vi "Idot Continuous Recorder.vi"(8 "Error In":errorcluster, 9 "New data file event":refnum<user-event>, 10 "Stop event":refnum<user-event>, 11 "Parameters":T1={"physical channels"="Dev1/ai0:7", "input terminal configuration"=10106, "Range"=10.0, "Sample rate"=1000000.0, "samples per channel"=220000, "Trigger source"="/Dev1/PFI0", "pretrigger samples per channel"=20000, "task"="", "Sample mode"=10178, "Retriggerable"=FALSE, "File Path"=path ""} {"Sample mode" items=["Finite Samples"=10178, "Continuous Samples"=10123, "Hardware Timed Single Point"=12522]; "Sample rate" format="%.2p"; "input terminal configuration" items=["default"=-1, "RSE"=10083, "NRSE"=10078, "Differential"=10106, "Pseudodifferential"=12529]}) -> (0 "Error Out":errorcluster)   [LabVIEW 2015]
uses:
  NI-DAQ/NI-DAQ digitizer parameters.ctl
  <resource>/objmgr/daqmx.rc
panel:
  out "Done":bool
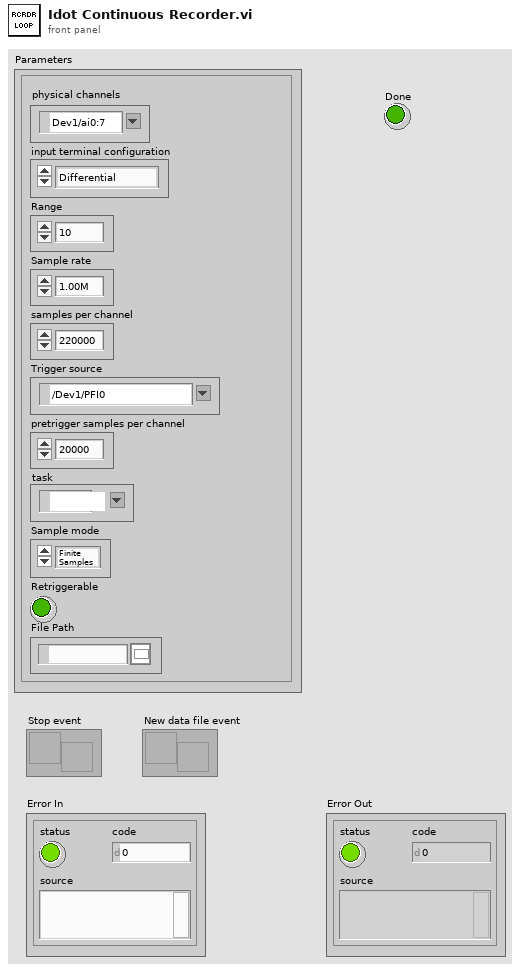
[diagram p1: front panel]
types:
  T1 = typedef "NI-DAQ digitizer parameters.ctl" = cluster{"physical channels":tag, "input terminal configuration":i32, "Range":dbl, "Sample rate":dbl, "samples per channel":i32, "Trigger source":tag, "pretrigger samples per channel":u32, "task":refnum<k21>, "Sample mode":i32, "Retriggerable":bool, "File Path":path}
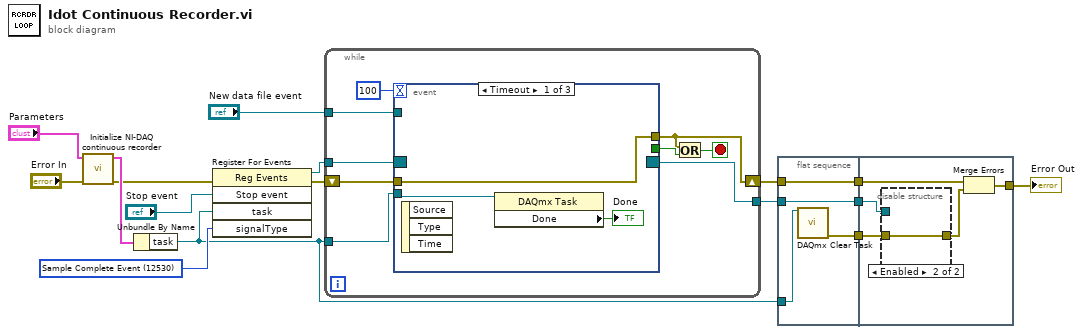
[diagram p0: block diagram]
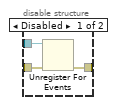
[diagram p2: hidden frame]
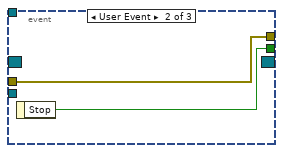
[diagram p3: hidden frame]
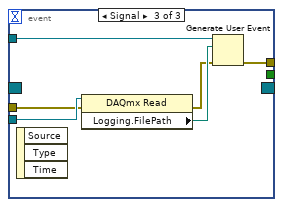
[diagram p4: hidden frame]
diagram:
  w6 = 12530 items=["Sample Complete Event"=12530, "Counter Output Event"=12494, "Change Detection Event"=12511, "Sample Clock"=12487] ("signalType")
  n1 = call "Initialize NI-DAQ continuous recorder.vi"("error in (no error)"="Error In", "Parameters"="Parameters") -> ("error out"=w13:errorcluster, "Parameters out"=w16:T1)  [unwired: 8 in]
  n2 = Unbundle By Name(w16) -> ("task"=w5:refnum<k21>)
  n3 = register-events(error in=w13, "Stop event", w5, w6) -> (reference out=w8:refnum<event-registration>, error out=w12:errorcluster)  [unwired: 1 in]
  n4 = while {
    tunnel: w8 -> [w25]
    shift-right: [w21] -> w10
    shift-left: w12 -> [w24]
    tunnel: [w20] -> w7
    tunnel: w5 -> [w18]
    tunnel: "New data file event" -> [w17]
    stop <- w23 stop-if-true
    n5 = event shown="[0] Timeout" {
      selector: w25 -> [_ _ _]
      dyn-events: [_ _ _] -> w20
      timeout: 100 -> [_ _ _]
      tunnel: w24 -> [w28 w29 w35]
      tunnel: [w28 w29 w31] -> w21
      tunnel: [_ w30 _] -> w22
      tunnel: w18 -> [w27 _ w36]
      tunnel: w17 -> [_ _ w34]
      event Timeout {
        n6 = event-data() -> ()  [unwired: 1 in, 3 out]
        n7 = property class="DAQmx Task"(reference=w27) -> ("Done"=→"Done":bool)  [unwired: 1 in, 2 out]
      }
      event User Event {
        n8 = event-data() -> ("Stop"=w30:bool)  [unwired: 1 in]
      }
      event Signal {
        n9 = event-data() -> ()  [unwired: 1 in, 3 out]
        n10 = property class="DAQmx Read"(reference=w36, error in=w35) -> (error out=w32:errorcluster, "Logging.FilePath"=w33:path)  [unwired: 1 out]
        n11 = Generate User Event(user event=w34, event data cluster=w33, error in=w32) -> (error out=w31:errorcluster)  [unwired: 1 in, 1 out]
      }
    }
    n12 = Or(x=w21, y=w22) -> (x .or. y?=w23:bool)
  }
  n13 = flat-sequence {
    tunnel: w7 -> [w39]
    tunnel: w5 -> [w38]
    tunnel: w10 -> [w40]
    tunnel: [w40] -> w3
    tunnel: [w37] -> w2
    tunnel: [w39] -> w1
    tunnel: [w44] -> w9
    tunnel: w3 -> [w45]
    tunnel: w2 -> [w41]
    tunnel: w1 -> [w43]
    frame #0 {
      n14 = call <vilib>:"DAQmx Clear Task.vi"("task in"=w38) -> ("error out"=w37:errorcluster)  [unwired: 14 in]
    }
    frame #1 {
      n15 = disable-structure shown="Enabled" {
        disable-tunnel: w43 -> [w48 _]
        disable-tunnel: [w47 w49] -> w42
        disable-tunnel: w41 -> [w46 w49]
        frame Disabled {
          n16 = Unregister For Events(event registration refnum=w48, error in=w46) -> (error out=w47:errorcluster)
        }
        frame Enabled {
        }
      }
      n17 = Merge Errors(w45, w42) -> (w44:errorcluster)
    }
  }
  "Error Out" <- w9
